vi "LINC Register Error.vi"(8 "error in (no error)":errorcluster, 11 "LINC session":refnum<class "LINC.lvclass">) -> (0 "error out":errorcluster, 3 "dup LINC session":refnum<class "LINC.lvclass">)   [LabVIEW 2018, in "STEPkgDriver_LINC.lvlib" / "LINC.lvclass"]
uses:
  LINC.lvclass
panel:
  in  "ERROR":errorcluster
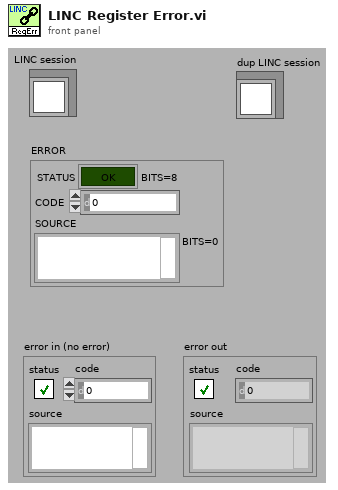
[diagram p1: front panel]
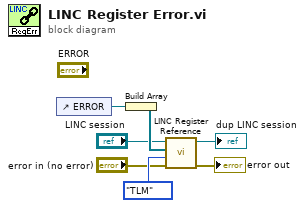
[diagram p0: block diagram]
diagram:
  n1 = control-ref of="ERROR"() -> (w4:refnum<vi>)
  n2 = Build Array(w4) -> (w3:refnum<vi>[])
  n3 = call "LINC Register Reference.vi"("error in (no error)"="error in (no error)", "type (CMD)"=enum16{"CMD", "TLM", "CMD_HDR", "TLM_HDR"}."TLM", "controls"=w3, "LINC session"="LINC session") -> ("error out"=→"error out":errorcluster, "dup LINC session"=→"dup LINC session":refnum<class "LINC.lvclass">)  [unwired: 6 in]
